vi "Set Text Message.vi"(8 "error in (no error)":errorcluster, 10 "Observable":refnum<class "Observable.lvclass">, 11 "Reverse Text in":refnum<class "Reverse Text.lvclass">) -> (0 "error out":errorcluster, 3 "Reverse Text out":refnum<class "Reverse Text.lvclass">)   [LabVIEW 2011, in "Reverse Text.lvclass"]
uses:
  Reverse Text.lvclass
  Observable/Observable.lvclass
  Reverse Text.lvclass/Reverse Text.ctl
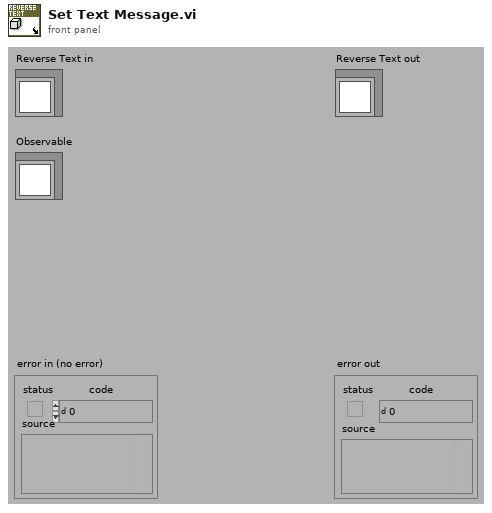
[diagram p1: front panel]
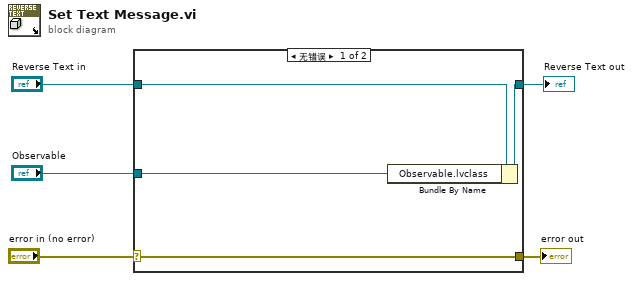
[diagram p0: block diagram]
diagram:
  n1 = case shown="无错误" "error in (no error)" {
    selector: "error in (no error)" -> [w9 w10]
    tunnel: [w9 w10] -> w2
    tunnel: [w7 w11] -> w4
    tunnel: "Reverse Text in" -> [w8 w11]
    tunnel: "Observable" -> [w6 _]
    frame No Error {
      n2 = Bundle By Name(cluster=w8, "Observable.lvclass"=w6) -> (w7:refnum<class "Reverse Text.lvclass">)
    }
    frame Error {
    }
  }
  "error out" <- w2
  "Reverse Text out" <- w4
